vi "Read Sigle int.vi"(8 "error in (no error)":errorcluster, 11 "Tags":string) -> (0 "error out":errorcluster, 2 "Data Byte":i16, 3 "Siemens Ctr out":T1)   [LabVIEW 2014]
uses:
  Simatic S7.lvlib
panel:
  in  "file path (dialog if empty)":path caption="文件路径 （空时为对话框）"
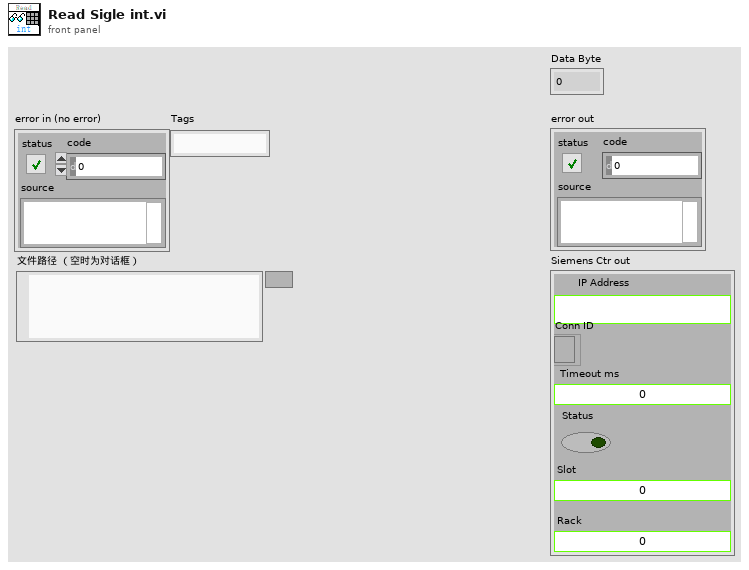
[diagram p1: front panel]
types:
  T1 = typedef "Simatic S7.lvlib/Siemens Ref.ctl" = cluster{"IP Address ":string, "Conn ID":refnum<k5>, "Timeout ms":i32, "Status":bool, "Slot":u16, "Rack":u16}
  T2 = typedef "Simatic S7.lvlib/Operation Siemens Ref.ctl" = enum16{"Init", "Add Ref", "Get Ref", "Set Error", "Close Close"}
  T3 = typedef "PLC Address.ctl" = cluster{"Address Areas":u8, "Data Type":enum8{"Bit", "Byte", "int", "Word", "Dint", "Dword", "Real", "String"}, "DB.No":u16, "Byte":u32, "Length":u16, "Item":u16}
  T4 = typedef "Semaphore RefNum" = refnum<k1>
  T5 = typedef "Simatic S7.lvlib/Op ip address.ctl" = enum16{"Init", "Add IP", "Get IP"}
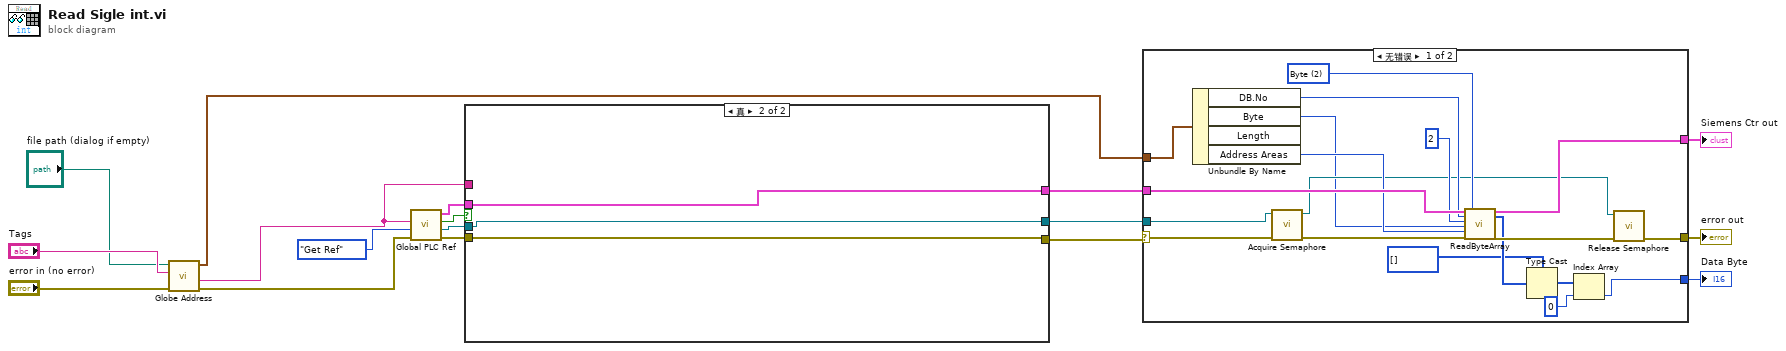
[diagram p0: block diagram]
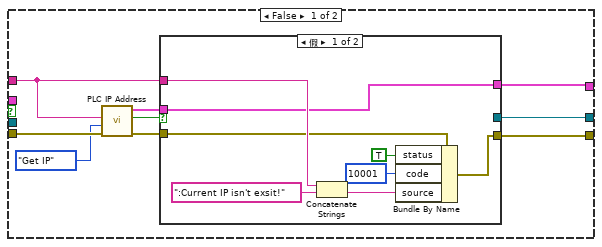
[diagram p3: hidden frame]
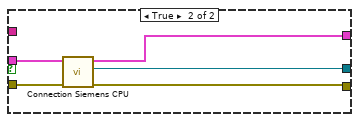
[diagram p4: hidden frame]
diagram:
  n1 = call "Globe Address.vi"("error in (no error)"="error in (no error)", "Tag"="Tags", "file path (dialog if empty)"="file path (dialog if empty)") -> ("error out"=w8:errorcluster, "IP"=w7:string, "ddress"=w5:T3)  [unwired: 5 in, 1 out]
  n2 = call "Global PLC Ref.vi"("error in (no error)"=w8, "Operation Siemens Ref"=Operation_Siemens_Ref."Get Ref", "IP Address"=w7) -> ("error out"=w15:errorcluster, "semaphore"=w13:T4, "Boolean"=w16:bool, "Siemens Ctr out"=w14:T1)  [unwired: 4 in, 1 out]
  n3 = case shown="真" w16 {
    tunnel: w15 -> [w26 w42]
    tunnel: w7 -> [w22 _]
    tunnel: [w20 w42] -> w12
    tunnel: [w19 w40] -> w11
    tunnel: [w18 w41] -> w10
    tunnel: w14 -> [_ w41]
    tunnel: w13 -> [_ w40]
    frame False {
      n4 = call "PLC IP Address.vi"("error in (no error)"=w26, "Operationip"=Op_ip_address."Get IP", "IP Address"=w22) -> ("error out"=w23:errorcluster, "Boolean"=w24:bool, "Siemens Ctr out"=w21:T1)  [unwired: 6 in]
      n5 = case shown="假" w24 {
        tunnel: w23 -> [w32 w39]
        tunnel: w22 -> [w33 _]
        tunnel: w21 -> [w27 w38]
        tunnel: [w28 w37] -> w20
        tunnel: [_ w36] -> w19
        tunnel: [w27 w35] -> w18
        frame False {
          n6 = Concatenate Strings(w33, ":Current IP isn't exsit!") -> (w30:string)
          n7 = Bundle By Name(cluster=w32, "status"=TRUE, "code"=10001, "source"=w30) -> (w28:errorcluster)
        }
        frame True {
          n8 = call "Connection Siemens CPU.vi"("error in (no error)"=w39, "Siemens Ctr in"=w38) -> ("error out"=w37:errorcluster, "semaphore"=w36:T4, "Siemens Ctr out"=w35:T1)  [unwired: 7 in]
        }
      }
    }
    frame True {
    }
  }
  n9 = case shown="无错误" w12 {
    selector: w12 -> [w61 w63]
    tunnel: w11 -> [w54 _]
    tunnel: w10 -> [w59 w62]
    tunnel: w5 -> [w58 _]
    tunnel: [w50 w63] -> w4
    tunnel: [w52 w62] -> w3
    tunnel: [w44 _] -> w1
    frame No Error {
      w57 = u8 2 items=["Boolen"=1, "Byte"=2] ("Bit/Byte")
      n10 = Unbundle By Name(w58) -> ("DB.No"=w56:u16, "Byte"=w48:u32, "Address Areas"=w53:u8)  [unwired: 1 out]
      n11 = call <vilib>:"Acquire Semaphore.vi"("error in (no error)"=w61, "semaphore"=w54) -> ("error out"=w60:errorcluster, "semaphore out"=w49:T4)  [unwired: 3 in, 1 out]
      n12 = call "ReadByteArray.vi"("Siemens Ctr"=w59, "# DB No."=w56, "#items"=u16 2, "Item offset [byte]"=w48, "Address Areas"=w53, "error in (no error)"=w60, "Bit/Byte"=w57) -> ("Siemens Ctr out"=w52:T1, "Byte Array"=w47:u8[], "error out"=w51:errorcluster)  [unwired: 10 in]
      n13 = Type Cast(type=i16[] [], x=w47) -> (*(type *) &x=w46:i16[])
      n14 = Index Array(array=w46, index=0) -> (element=w44:i16)
      n15 = call <vilib>:"Release Semaphore.vi"("error in (no error)"=w51, "semaphore"=w49) -> ("error out"=w50:errorcluster)  [unwired: 4 in, 1 out]
    }
    frame Error {
    }
  }
  "error out" <- w4
  "Siemens Ctr out" <- w3
  "Data Byte" <- w1
